vi "local ODMR B sweep.vi"() -> ()   [LabVIEW 2012]
uses:
  <vilib>/Utility/file.llb/Read From Spreadsheet File (DBL).vi
  <vilib>/Utility/file.llb/Write To Spreadsheet File (DBL).vi
  <vilib>/express/express arith-compare/Formula/XNode/ExpressFormulaBlockNode.xnode
panel:
  in  "freq width":dbl
  in  "Voltage Step":dbl
  in  "file path (dialog if empty)":path
  in  "Z-track?":bool
  in  "Z Pos":dbl=52.1
  in  "Y pos":dbl=25.0
  in  "X Pos":dbl=128.0
  in  "Y Parameters":T1={"Number of Y Steps"=200, "Max Y (V)"=2.0, "Min Y (V)"=-2.0}
  in  "X":T2={"Number of X Steps"=200, "Max X (V)"=2.0, "Min X (V)"=-2.0}
  in  "ODMR res file":path
  out "ODMR freq":ext
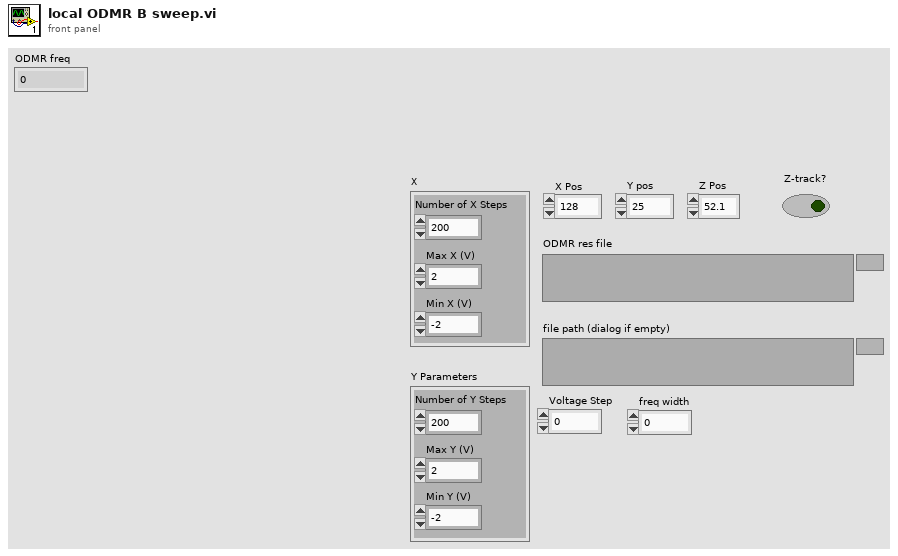
[diagram p1: front panel]
types:
  T1 = cluster{"Number of Y Steps":i32, "Max Y (V)":dbl, "Min Y (V)":dbl}
  T2 = cluster{"Number of X Steps":i32, "Max X (V)":dbl, "Min X (V)":dbl}
  T3 = cluster{"GPIB address 2":string, "resolution (10 Hz:2) 2":i32, "band (1-26.5:2) 2":i32, "Freq max":ext, "Start Voltage":dbl, "Voltage Step":dbl, "rate":dbl, "samples per channel":i32}
  T4 = cluster{"RS232 settings":cluster{"Portnumber":i32, "Baudrate":u16}, "X Parameters":cluster{"Number of X Steps":i32, "Max X (V)":dbl, "Min X (V)":dbl}, "Y Parameters":cluster{"Number of Y Steps":i32, "Max Y (V)":dbl, "Min Y (V)":dbl}, "X Pos":dbl, "Y Pos":dbl, "Z Pos":dbl, "Tracking interval":dbl}
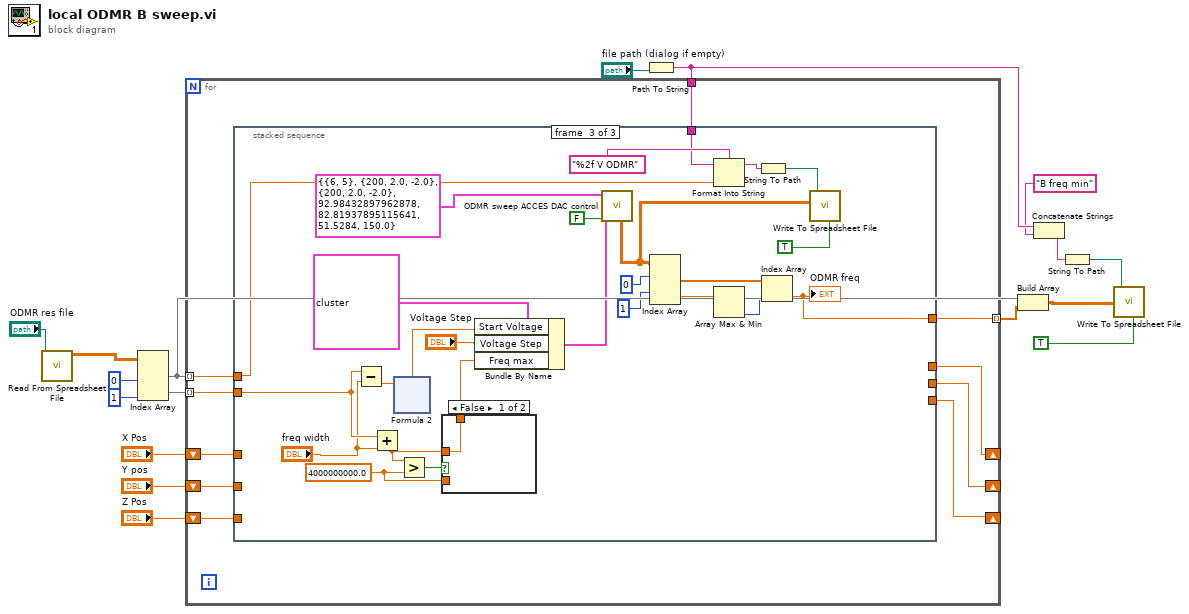
[diagram p0: block diagram]
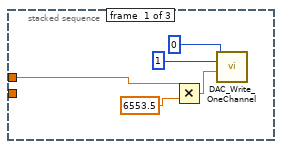
[diagram p2: hidden frame]
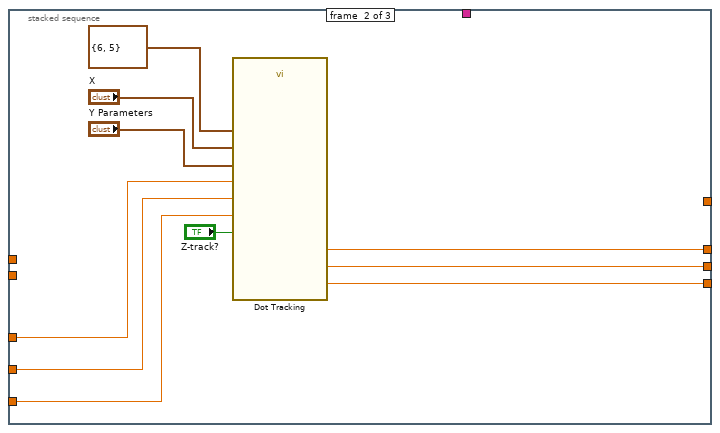
[diagram p3: hidden frame]
diagram:
  n1 = call-poly <vilib>:"Read From Spreadsheet File.vi"("file path (dialog if empty)"="ODMR res file") -> ("all rows"=w15:dbl[][])  [unwired: 6 in, 4 out]
  n2 = Index Array(array=w15, index (col) #1=0 ("disabled index (col)"), index (col) #2=1 ("index (col)")) -> (element #1=w8:dbl[], element #2=w13:dbl[])  [unwired: 2 in]
  n3 = Path To String(path="file path (dialog if empty)") -> (string=w4:string)
  n4 = for {
    tunnel: w8 -> [w27] mode=indexing
    tunnel: w13 -> [w26] mode=indexing
    shift-right: [w20] -> _
    shift-left: "Z Pos" -> [w23]
    shift-right: [w21] -> _
    shift-left: "Y pos" -> [w24]
    shift-right: [w22] -> _
    shift-left: "X Pos" -> [w25]
    tunnel: [w19] -> w9 mode=indexing
    tunnel: w4 -> [w18]
    n5 = stacked-sequence {
      tunnel: w27 -> [w29 _ w53]
      tunnel: w26 -> [_ _ w57]
      tunnel: w25 -> [_ w39 _]
      tunnel: w24 -> [_ w38 _]
      tunnel: w23 -> [_ w37 _]
      tunnel: [_ w36 _] -> w22
      tunnel: [_ w35 _] -> w21
      tunnel: [_ w34 _] -> w20
      tunnel: [_ _ w56] -> w19
      tunnel: w18 -> [_ _ w51]
      frame #0 {
        n6 = Multiply(x=w29, y=6553.5) -> (x*y=w32:dbl)
        n7 = call "DAC_Write_OneChannel.vi"("Value"=w32, "Channel"=u16 1, "DeviceIndex"=u64 0) -> ()  [unwired: 7 in, 2 out]
      }
      frame #1 {
        n8 = call "Dot Tracking.vi"("X"="X", "Y Parameters"="Y Parameters", "RS232 settings"=cluster{"Portnumber":i32, "Baudrate":u16} {"Portnumber"=6, "Baudrate"=5}, "X Pos"=w39, "Y pos"=w38, "Z Pos"=w37, "Z-track?"="Z-track?") -> ("X Position"=w36:dbl, "Y Position"=w35:dbl, "Z Position"=w34:dbl)  [unwired: 2 in, 4 out]
      }
      frame #2 {
        w46 = 4000000000.0 ("y")
        n9 = Subtract(x=w57, y="freq width") -> (x-y=w64:dbl)
        n10 = Add(x=w57, y="freq width") -> (x+y=w47:dbl)
        n11 = xnode "Formula 2"("X1"=w64) -> ("Result"=w65:dbl)  [unwired: 1 in, 1 out]
        n12 = Greater?(x=w47, y=w46) -> (0:w48:bool)
        n13 = case shown="False" w48 {
          tunnel: w47 -> [w69 _]
          tunnel: w46 -> [_ w70]
          tunnel: [w69 w70] -> w45
          frame False {
          }
          frame True {
          }
        }
        n14 = Bundle By Name(cluster=T3 {"GPIB address 2"="19", "resolution (10 Hz:2) 2"=2, "band (1-26.5:2) 2"=2, "Freq max"=4000000000.0, "Start Voltage"=0.0, "Voltage Step"=0.02, "rate"=100.0, "samples per channel"=200} ("Freq Sweep Cluster"), "Start Voltage"=w65, "Voltage Step"="Voltage Step", "Freq max"=w45) -> (w66:T3)
        n15 = call "ODMR sweep ACCES DAC control.vi"("Save?"=FALSE, "Freq Sweep Cluster"=w66, "Dot Tracking Cluster"=T4 {"RS232 settings"={"Portnumber"=6, "Baudrate"=5}, "X Parameters"={"Number of X Steps"=200, "Max X (V)"=2.0, "Min X (V)"=-2.0}, "Y Parameters"={"Number of Y Steps"=200, "Max Y (V)"=2.0, "Min Y (V)"=-2.0}, "X Pos"=92.98432897962878, "Y Pos"=82.81937895115641, "Z Pos"=51.5284, "Tracking interval"=150.0}) -> ("appended array"=w55:ext[][])  [unwired: 4 in, 4 out]
        n16 = Index Array(array=w55, index (row) #1=0 ("disabled index (col)"), index (row) #2=1 ("index (col)")) -> (element #1=w61:ext[], element #2=w62:ext[])  [unwired: 2 in]
        n17 = Format Into String(format string="%2f V ODMR", initial string=w51, w53) -> (resulting string=w50:string)  [unwired: 1 in, 1 out]
        n18 = Array Max & Min(array=w62) -> (min index (indices)=w60:i32)  [unwired: 3 out]
        n19 = String To Path(string=w50) -> (path=w49:path)
        n20 = Index Array(array=w61, index=w60) -> (element=w56:ext)
        "ODMR freq" <- w56
        n21 = call-poly <vilib>:"Write To Spreadsheet File.vi"("transpose? (no:F)"=TRUE, "2D data"=w55, "file path (dialog if empty)"=w49) -> ()  [unwired: 5 in, 1 out]
      }
    }
  }
  n22 = Build Array(w8, w9) -> (w7:ext[][])
  n23 = Concatenate Strings(w4, "B freq min" ("string")) -> (w2:string)
  n24 = String To Path(string=w2) -> (path=w1:path)
  n25 = call-poly <vilib>:"Write To Spreadsheet File.vi"("transpose? (no:F)"=TRUE, "2D data"=w7, "file path (dialog if empty)"=w1) -> ()  [unwired: 5 in, 1 out]
